vi "emi_Start Loop.vi"   [LabVIEW 2010]
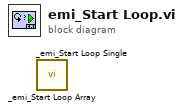
[diagram p0: block diagram]
diagram:
  n1 = call "_emi_Start Loop Array.vi"() -> ()  [unwired: 13 in, 3 out]
  n2 = call "_emi_Start Loop Single.vi"() -> ()  [unwired: 13 in, 3 out]
